vi "录屏工具.vi"() -> ()   [LabVIEW 2025]
uses:
  user32.dll
panel:
  in  "暂停":bool=TRUE
  out "Image Out":T1(plugin-control)
  in  "开始":bool
  in  "每秒播放帧数":u32=10
  out "用时":dbl
  out "Filter Names":string[](array[string])
  out "格式":string
  in  "格式更改":i32=6
  in  "?":bool
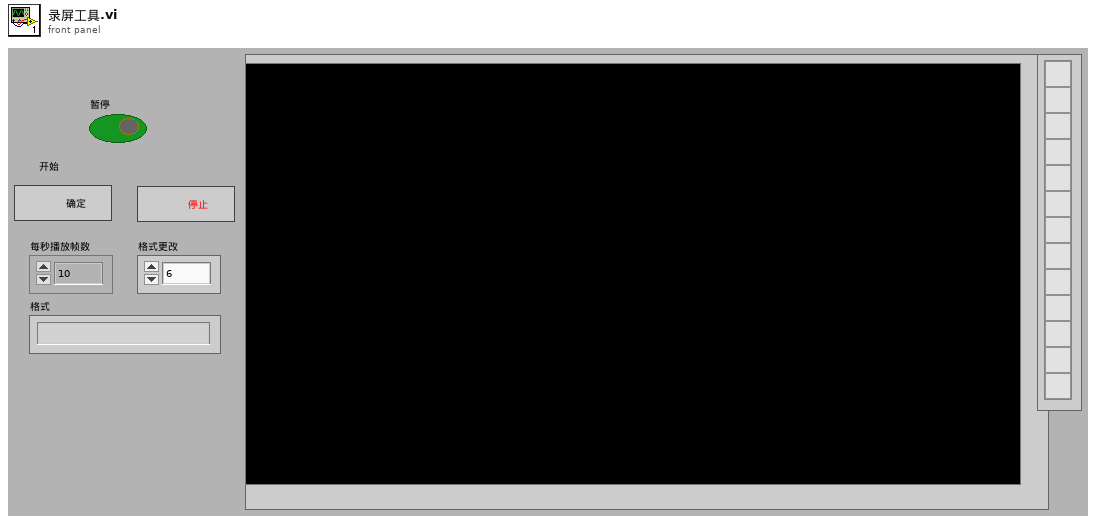
[diagram p1: front panel]
types:
  T1 = typedef "IMAQ Image.ctl" = refnum<image>
  T2 = enum32{"Invalid", "Standard", "Closed", "Hidden", "Minimized", "Maximized"}
  T3 = typedef "AviRefnum.ctl" = refnum<k1>
  T4 = typedef "Image Type" = u32
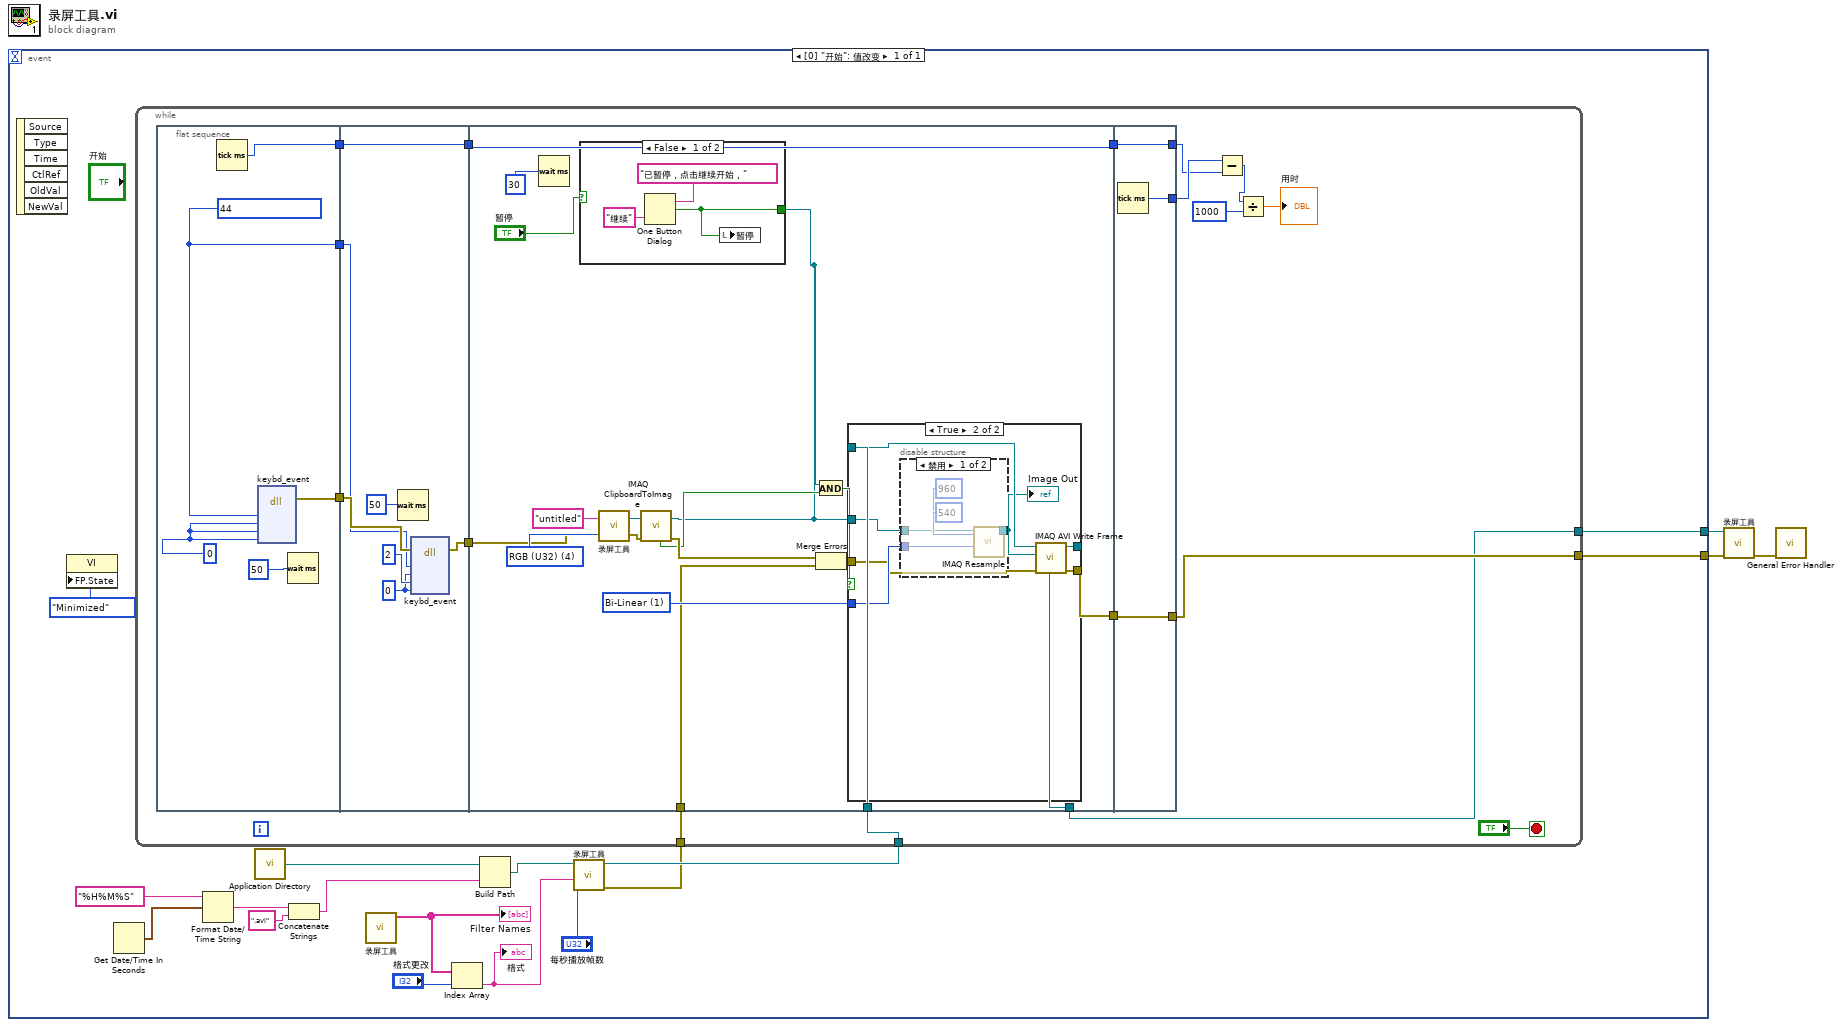
[diagram p0: block diagram]
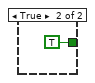
[diagram p2: hidden frame]
diagram:
  n1 = event shown="[0] \"开始\": 值改变" {
    selector: _ -> [_]
    dyn-events: _ -> [_]
    timeout: _ -> [_]
    tunnel: [w6] -> w2
    tunnel: [w5] -> w1
    event "开始": Value Change {
      n2 = event-data() -> ()  [unwired: 1 in, 6 out]
      n3 = property class="VI"("FP.State"=T2."Minimized" ("前面板窗口:状态")) -> ()  [unwired: 2 in, 2 out]
      n4 = Get Date/Time In Seconds() -> (seconds since 1Jan1904=w14:timestamp)
      n5 = Format Date/Time String(time format string (%c)="%H%M%S" ("时间格式字符串(%c)"), seconds (now)=w14) -> (date/time string=w11:string)  [unwired: 1 in]
      n6 = call <vilib>:"Application Directory.vi"() -> ("Application Directory"=w4:path)
      n7 = Concatenate Strings(w11, ".avi" ("字符串")) -> (w10:string)
      n8 = call "录屏工具.vi"() -> ("Filter Names"=w17:string[])  [unwired: 10 in, 1 out]
      "Filter Names" <- w17
      n9 = Index Array(array=w17, index="格式更改") -> (element=w15:string)
      "格式" <- w15
      n10 = Build Path(base path=w4, name or relative path=w10) -> (appended path=w19:path)
      n11 = call "录屏工具.vi"("Compression Filter"=w15, "Frames Per Second"="每秒播放帧数", "AVI Path"=w19) -> ("error out"=w8:errorcluster, "Avi Refnum"=w18:T3)  [unwired: 7 in]
      n12 = while {
        tunnel: w18 -> [w35]
        tunnel: w8 -> [w22]
        tunnel: [w21] -> w6
        tunnel: [w20] -> w5
        stop <- "?" stop-if-true
        n13 = flat-sequence {
          tunnel: [w41] -> w31
          tunnel: [w39] -> w25
          tunnel: [w38] -> w24
          tunnel: [w47] -> w32
          tunnel: w31 -> [w47]
          tunnel: w25 -> [w45]
          tunnel: w24 -> [w44]
          tunnel: [w42] -> w23
          tunnel: w35 -> [w66]
          tunnel: [w65] -> w34
          tunnel: [w64] -> w33
          tunnel: w32 -> [w64]
          tunnel: [w62] -> w20
          tunnel: w23 -> [w57]
          tunnel: w22 -> [w54]
          tunnel: [w88] -> w21
          tunnel: w34 -> [w88]
          tunnel: [w87] -> w29
          tunnel: w33 -> [w87]
          tunnel: [w86] -> w30
          frame #0 {
            w40 = u8 0 ("bScan")
            w38 = u16 44 ("Extended Virtual Key List")
            n14 = Tick Count (ms)() -> (millisecond timer value=w41:u32)
            n15 = dll-call lib="user32.dll" fn="keybd_event"("bVk"=w38, "bScan"=w40, "dwFlags"=w40, "dwExtraInfo"=w40) -> (error out=w39:errorcluster)  [unwired: 4 in, 5 out]
            n16 = Wait (ms)(milliseconds to wait=u32 50 ("等待时间（毫秒）")) -> ()  [unwired: 1 out]
          }
          frame #1 {
            w46 = u8 0 ("bScan")
            n17 = Wait (ms)(milliseconds to wait=u32 50 ("等待时间（毫秒）")) -> ()  [unwired: 1 out]
            n18 = dll-call lib="user32.dll" fn="keybd_event"(error in=w45, "bVk"=w44, "bScan"=w46, "dwFlags"=u32 2, "dwExtraInfo"=w46) -> (error out=w42:errorcluster)  [unwired: 4 in, 4 out]
          }
          frame #2 {
            w58 = T4 4 items=["Grayscale (U8)", "Grayscale (I16)", "Grayscale (SGL)", "Complex (CSG)", "RGB (U32)", "HSL (U32)", "RGB (U64)", "Grayscale (U16)"] ("Image Type")
            w61 = u32 1 items=["Zero Order", "Bi-Linear", "Quadratic", "Cubic Spline"] ("Interpolation Type")
            n19 = Wait (ms)(milliseconds to wait=u32 30 ("等待时间（毫秒）")) -> ()  [unwired: 1 out]
            n20 = call "录屏工具.vi"("Image Name"="untitled", "Image Type"=w58, "error in (no error)"=w57) -> ("New Image"=w60:T1, "error out"=w56:errorcluster)  [unwired: 2 in]
            n21 = call "IMAQ ClipboardToImage"("error in (no error)"=w56, "Image"=w60) -> ("Clipboard has an image?"=w52:bool, "error out"=w55:errorcluster, "Image Out"=w49:T1)  [unwired: 3 in, 1 out]
            n22 = case shown="False" "暂停" {
              tunnel: w49 -> [w67 TRUE ("true")]
              frame False {
                n23 = One Button Dialog(message="已暂停，点击继续开始，" ("消息"), button name ("OK")="继续" ("按钮名称（“确定”）")) -> (true=w67:bool)
                n24 = local write "暂停"(w67) -> ()
              }
              frame True {
              }
            }
            n25 = And(x=w49, y=w52) -> (x .and. y?=w51:bool)
            n26 = Merge Errors(w55, w54) -> (w53:errorcluster)
            n27 = case shown="True" w51 {
              tunnel: w66 -> [w72 w79]
              tunnel: w49 -> [_ w75]
              tunnel: [w72 w77] -> w62
              tunnel: [w71 w78] -> w65
              tunnel: w61 -> [_ w76]
              tunnel: w53 -> [w71 w73]
              frame False {
              }
              frame True {
                n28 = disable-structure shown="禁用" {
                  disable-tunnel: w76 -> [w82 _]
                  disable-tunnel: w75 -> [w81 w85]
                  disable-tunnel: [w80 w85] -> w74
                  frame Disabled {
                    n29 = call "IMAQ Resample"("X Resolution"=960, "Y Resolution"=540, "Interpolation Type"=w82, "Image Src"=w81) -> ("Image Dst Out"=w80:T1)  [unwired: 6 in, 1 out]
                  }
                  frame Enabled {
                  }
                }
                "Image Out" <- w74
                n30 = call "IMAQ AVI Write Frame"("error in (no error)"=w73, "Image"=w74, "Avi Refnum"=w79) -> ("error out"=w78:errorcluster, "Avi Refnum (duplicate)"=w77:T3)  [unwired: 7 in]
              }
            }
          }
          frame #3 {
            n31 = Tick Count (ms)() -> (millisecond timer value=w86:u32)
          }
        }
        n32 = Subtract(x=w30, y=w29) -> (x-y=w28:u32)
        n33 = Divide(x=w28, y=u32 1000) -> (x/y=→"用时":dbl)
      }
    }
  }
  n34 = call "录屏工具.vi"("error in (no error)"=w2, "Avi Refnum"=w1) -> ("error out"=w3:errorcluster)  [unwired: 9 in]
  n35 = call <vilib>:"General Error Handler.vi"("error in (no error)"=w3) -> ()  [unwired: 10 in, 5 out]
